vi "Set panel size and  place center.vi"(0 "VI引用句柄":refnum<vi>, 1 "Close Reference (false)":bool, 2 "FP.WinOrigin in(H & V)":cluster{"Horizontal":i16, "Vertical":i16}, 5 "Panel Width":i32, 7 "Panel Height":i32, 9 "FP.Origin in(H & V)":cluster{"Horizontal":i16, "Vertical":i16}, 11 "error in (no error)":errorcluster, 12 "Set (false)":bool) -> (4 "Application or VI Refnum":refnum<vi>, 15 "error out":errorcluster)   [LabVIEW 2016]
doc: "This VI is used to set the panel size and plce it in the center of the window current"
uses:
  <vilib>/Utility/miscctls.llb/LVRectTypeDef.ctl
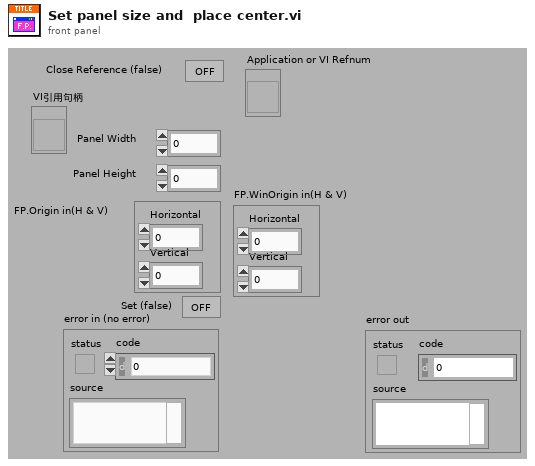
[diagram p1: front panel]
types:
  T1 = typedef "LVRectTypeDef.ctl" = cluster{"Left":i16, "Top":i16, "Right":i16, "Bottom":i16}
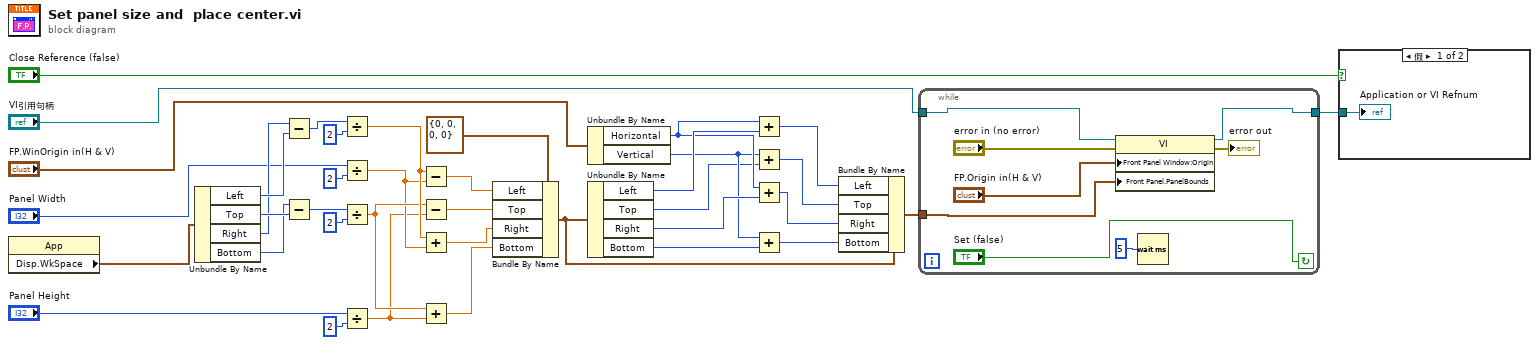
[diagram p0: block diagram]
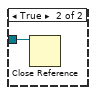
[diagram p2: hidden frame]
diagram:
  n1 = property class="App"() -> ("Disp.WkSpace"=w3:T1)  [unwired: 2 in, 2 out]
  n2 = Unbundle By Name(w3) -> ("Left"=w38:i16, "Top"=w37:i16, "Right"=w36:i16, "Bottom"=w35:i16)
  n3 = Subtract(x=w36, y=w38) -> (x-y=w34:i16)
  n4 = Subtract(x=w35, y=w37) -> (x-y=w32:i16)
  n5 = Divide(x=w34, y=i16 2) -> (x/y=w26:dbl)
  n6 = Divide(x="Panel Width", y=2) -> (x/y=w24:dbl)
  n7 = Divide(x=w32, y=i16 2) -> (x/y=w25:dbl)
  n8 = Divide(x="Panel Height", y=2) -> (x/y=w23:dbl)
  n9 = Subtract(x=w26, y=w24) -> (x-y=w22:dbl)
  n10 = Subtract(x=w25, y=w23) -> (x-y=w20:dbl)
  n11 = Add(x=w26, y=w24) -> (x+y=w19:dbl)
  n12 = Add(x=w25, y=w23) -> (x+y=w21:dbl)
  n13 = Bundle By Name(cluster=T1 {"Left"=0, "Top"=0, "Right"=0, "Bottom"=0} ("显示:主工作区"), "Left"=w22, "Top"=w20, "Right"=w19, "Bottom"=w21) -> (w15:T1)
  n14 = Unbundle By Name("FP.WinOrigin in(H & V)") -> ("Horizontal"=w11:i16, "Vertical"=w7:i16)
  n15 = Unbundle By Name(w15) -> ("Left"=w13:i16, "Top"=w4:i16, "Right"=w10:i16, "Bottom"=w6:i16)
  n16 = Add(x=w11, y=w13) -> (x+y=w12:i16)
  n17 = Add(x=w7, y=w4) -> (x+y=w8:i16)
  n18 = Add(x=w11, y=w10) -> (x+y=w9:i16)
  n19 = Add(x=w7, y=w6) -> (x+y=w5:i16)
  n20 = Bundle By Name(cluster=w15, "Left"=w12, "Top"=w8, "Right"=w9, "Bottom"=w5) -> (w2:T1)
  n21 = while {
    tunnel: [w40] -> w17
    tunnel: "VI引用句柄" -> [w39]
    tunnel: w2 -> [w41]
    stop <- "Set (false)" continue-if-true
    n22 = property class="VI"(reference=w39, error in="error in (no error)", "Front Panel Window:Origin"="FP.Origin in(H & V)", "Front Panel.PanelBounds"=w41) -> (reference out=w40:refnum<vi>, error out=→"error out":errorcluster)
    n23 = Wait (ms)(milliseconds to wait=u32 5) -> ()  [unwired: 1 out]
  }
  n24 = case shown="假" "Close Reference (false)" {
    tunnel: w17 -> [w47 w48]
    frame False {
      "Application or VI Refnum" <- w47
    }
    frame True {
      n25 = Close Reference(reference=w48) -> ()  [unwired: 1 in, 1 out]
    }
  }
